vi "HIOKI PW3390 ESR.vi"(8 "error in (no error)":errorcluster, 11 "VISA Resource":refnum<visa-resource-name>) -> (0 "error out":errorcluster, 1 "Bits Set":bool[](array[boolean]), 2 "Output Value":u8, 3 "VISA Resource out":refnum<visa-resource-name>)   [LabVIEW 2018]
doc: "Returns and clears the contents of the event register.\n\n<B>Note</B>\nbit7(PON): Power On Flag\nTurns to 1 when power is switched on or when power is returned after a blackout.\nbit6(URQ): User Request\nNot available in the PW3390.\nbit5(CME): Command Error\n (Ignores commands up to the message terminator)\nTurns to 1 when there are syntactical and command errors in the received commands.\nEWhen there is an error in the program header\nEWhen the data value is different from the specified value\nEWhen the data type is different from the specified type\n\nbit4(EXE): Execution error\nTurns to 1 when the command cannot be executed for whatever reason.\nEWhen the specified data is outside the set range \nEWhen the specified data cannot be set\nEWhen another function is in operation and the command cannot be executed (holding, integrating, etc.) \n\nbit3(DDE): Device-dependent error\nTurns to 1 when the command cannot be executed due to causes other than a command error, query error or execution error.\nEWhen there is an internal problem and the command could not be executed\n\nbit2(QYE): Query error\nTurns to 1 when the error is detected by the output cue control part.\nEWhen the data inundated the output cue\n\nbit1(RQC): Request for controller right\nNot available in the PW3390.\n\nbit0(OPC): Operation completed\nNot available in the PW3390."
panel:
  # "0"
  # "1"
  # "2"
  # "3"
  # "4"
  # "5"
  # "6"
  # "7"
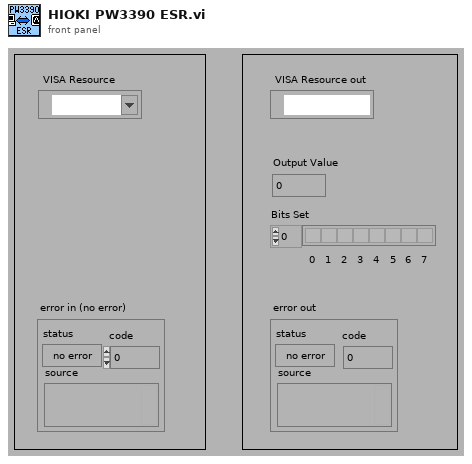
[diagram p1: front panel]
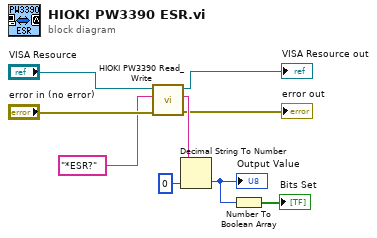
[diagram p0: block diagram]
diagram:
  n1 = call "HIOKI PW3390 Read_Write.vi"("error in (no error)"="error in (no error)", "data in"="*ESR?", "VISA Resource"="VISA Resource") -> ("error out"=→"error out":errorcluster, "data out"=w6:string, "VISA Resource out"=→"VISA Resource out":refnum<visa-resource-name>)  [unwired: 6 in]
  n2 = Decimal String To Number(string=w6, default (0L)=u8 0 ("デフォルト (0L)")) -> (number=w4:u8)  [unwired: 1 in, 1 out]
  "Output Value" <- w4
  n3 = Number To Boolean Array(number=w4) -> (Boolean array=→"Bits Set":bool[])
